vi "open_AnalysisWindow_dyn.vi"(8 "error in (no error)":errorcluster, 11 "Analysis in":refnum<class "Analysis.lvclass">) -> (0 "error out":errorcluster)   [LabVIEW 2015]
doc: "opens the AnalysisWindow dynamically"
uses:
  MSControl/Classes/Analysis/Analysis.lvclass
panel:
  out "appended path":path
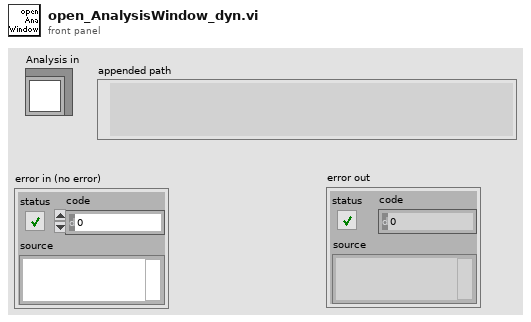
[diagram p1: front panel]
types:
  T1 = enum32{"Invalid", "Standard", "Closed", "Hidden", "Minimized", "Maximized"}
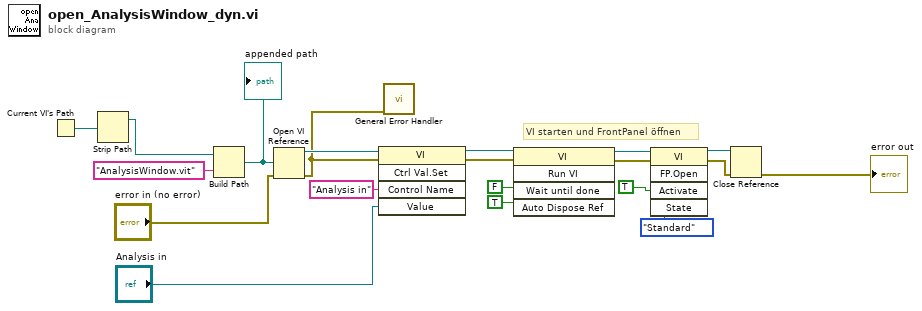
[diagram p0: block diagram]
diagram:
  # "VI starten und FrontPanel öffnen"
  n1 = Current VI's Path() -> (path=w5:path)
  n2 = Strip Path(path=w5) -> (stripped path=w3:path)  [unwired: 1 out]
  n3 = Build Path(base path=w3, name or relative path="AnalysisWindow.vit") -> (appended path=w4:path)
  "appended path" <- w4
  n4 = Open VI Reference(vi path=w4, error in (no error)="error in (no error)") -> (vi reference=w9:refnum<vi>, error out=w1:errorcluster)  [unwired: 4 in]
  n5 = invoke class="VI" method="Ctrl Val.Set"(reference=w9, error in=w1, "Control Name"="Analysis in", "Value"="Analysis in") -> (reference out=w8:refnum<vi>, error out=w7:errorcluster)  [unwired: 1 in, 3 out]
  n6 = call <vilib>:"General Error Handler.vi"("error in (no error)"=w1) -> ()  [unwired: 10 in, 5 out]
  n7 = invoke class="VI" method="Run VI"(reference=w8, error in=w7, "Wait until done"=FALSE, "Auto Dispose Ref"=TRUE) -> (reference out=w18:refnum<vi>, error out=w17:errorcluster)  [unwired: 1 in, 3 out]
  n8 = invoke class="VI" method="FP.Open"(reference=w18, error in=w17, "Activate"=TRUE, "State"=T1."Standard") -> (reference out=w14:refnum<vi>, error out=w13:errorcluster)  [unwired: 1 in, 3 out]
  n9 = Close Reference(reference=w14, error in (no error)=w13) -> (error out=→"error out":errorcluster)
